vi "Spin Shooter2 (Auto).vi"(10 "RPM (1900)":dbl=1900.0, 11 "Execute?":bool) -> (2 "Numeric":i32, 3 "Done":bool)   [LabVIEW 2012]
uses:
  Globals/Tachometer.vi
  Globals/Motors.vi
  <vilib>/addons/control/pid/pid.llb/PID (DBL).vi
  <vilib>/addons/control/pid/NI_PID_pid.lvlib
panel:
  out "Motor Out":dbl
  in  "Shooter Wheel PID gains":T1={"proportional gain (Kc)"=0.03, "integral time (Ti, min)"=0.0, "derivative time (Td, min)"=0.0} {"derivative time (Td, min)" format="%.3f"; "integral time (Ti, min)" format="%.3f"; "proportional gain (Kc)" format="%.3f"}
  in  "Shooter Limits":cluster{"output high":dbl, "output low":dbl}={"output high"=1.0, "output low"=0.0} {"output low" format="%.2f"; "output high" format="%.2f"}
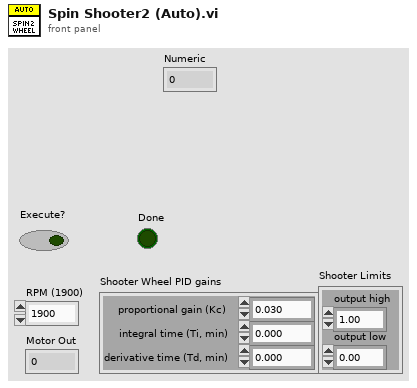
[diagram p1: front panel]
types:
  T1 = cluster{"proportional gain (Kc)":dbl, "integral time (Ti, min)":dbl, "derivative time (Td, min)":dbl}
  T2 = typedef "WPI_MotorControlDeviceRef.ctl" = cluster{"DeviceStatus":errorcluster, "Type":enum16{"PWM", "CAN"}, "PWM":cluster{"Digital Module":T3, "PWM Channel":T4, "DeadBand":T5}, "CAN":cluster{"Device Number":u8, "Control Mode":T6, "Semaphore":T7, "Max Vout":dbl}, "Invert":bool, "TransformRef":T8, "InvTransformRef":T8}
  T3 = typedef "FPGA_TypedefDigitalModule.ctl" = enum16{"Digital Module 1", "Digital Module 2"}
  T4 = typedef "FPGA_DIOPWMChannel.ctl" = enum8{"PWM 1", "PWM 2", "PWM 3", "PWM 4", "PWM 5", "PWM 6", "PWM 7", "PWM 8", "PWM 9", "PWM 10", "Invalid"}
  T5 = typedef "WPI_PWMDeadband.ctl" = cluster{"Name":string, "maxPositivePwm":i32, "minPositivePwm":i32, "centerPwm":i32, "maxNegativePwm":i32, "minNegativePwm":i32, "angularRange":u16}
  T6 = typedef "WPI_CANJaguar_ControlMode.ctl" = enum8{"Percent VBus", "Current", "Speed", "Position", "Voltage"}
  T7 = typedef "Semaphore RefNum" = refnum<k1>
  T8 = typedef "WPI_PWMTransform_ConPane.ctl" = refnum<vi>
  T9 = typedef "WPI_CounterDevRef.ctl" = cluster{"DevStatus":errorcluster, "CntIndex":T10}
  T10 = typedef "FPGA_CounterCtrSystemIndex.ctl" = enum8{"Ctr 0", "Ctr 1", "Ctr 2", "Ctr 3", "Ctr 4", "Ctr 5", "Ctr 6", "Ctr 7", "Invalid"}
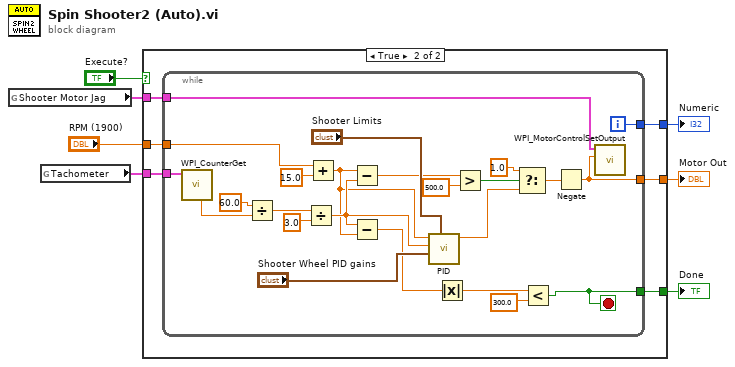
[diagram p0: block diagram]
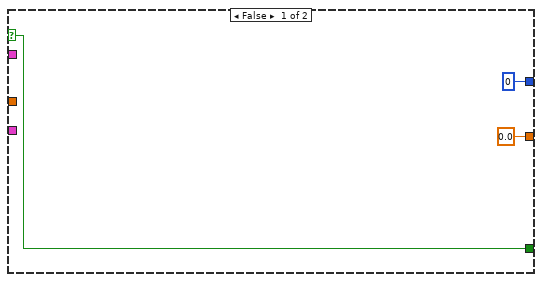
[diagram p2: hidden frame]
diagram:
  n1 = global read "Motors.vi" "Shooter Motor Jag"() -> (w2:T2)
  n2 = global read "Tachometer.vi" "Tachometer"() -> (w4:T9)
  n3 = case shown="True" "Execute?" {
    selector: "Execute?" -> [w10 _]
    tunnel: [w10 w11] -> w7
    tunnel: [0.0 w16] -> w5
    tunnel: w4 -> [_ w15]
    tunnel: "RPM (1900)" -> [_ w14]
    tunnel: w2 -> [_ w13]
    tunnel: [0 w12] -> w1
    frame False {
    }
    frame True {
      n4 = while {
        tunnel: w15 -> [w36]
        tunnel: w13 -> [w33]
        tunnel: [w29] -> w16
        tunnel: w14 -> [w24]
        tunnel: [w20] -> w12
        tunnel: [w17] -> w11
        i -> [w20]
        stop <- w17 stop-if-true
        n5 = call <vilib>:"WPI_CounterGet.vi"("CounterDevRef in"=w36) -> ("Period (sec)"=w38:dbl)  [unwired: 5 in, 5 out]
        n6 = Divide(x=60.0, y=w38) -> (x/y=w40:dbl)
        n7 = Divide(x=w40, y=3.0) -> (x/y=w23:dbl)
        n8 = Add(x=w24, y=15.0) -> (x+y=w22:dbl)
        n9 = Subtract(x=w22, y=w23) -> (x-y=w26:dbl)
        n10 = Subtract(x=w23, y=w22) -> (x-y=w21:dbl)
        n11 = call-poly <vilib>:"PID.vi"("output range"="Shooter Limits", "PID gains"="Shooter Wheel PID gains", "process variable"=w23, "setpoint"=w22) -> ("output"=w31:dbl)  [unwired: 6 in, 1 out]
        n12 = Absolute Value(x=w21) -> (abs(x)=w19:dbl)
        n13 = Greater?(x=w26, y=500.0) -> (0:w28:bool)
        n14 = Select(t=1.0, s=w28, f=w31) -> (s? t:f=w30:dbl)
        n15 = Less?(x=w19, y=300.0) -> (x < y?=w17:bool)
        n16 = Negate(x=w30) -> (-x=w29:dbl)
        n17 = call <vilib>:"WPI_MotorControlSetOutput.vi"("Output"=w29, "MotorControlDevRef"=w33) -> ()  [unwired: 7 in, 3 out]
      }
    }
  }
  "Done" <- w7
  "Motor Out" <- w5
  "Numeric" <- w1
